vi "Write to CSV Test.vi"(8 "Error In":errorcluster) -> (0 "Error Out":errorcluster)   [LabVIEW 2023, in "Test.lvlib"]
uses:
  Test.lvlib
  <vilib>/addons/_JKI Toolkits/Caraya/classes/Assert/Assert Equal Value_Variant.vi
  <vilib>/addons/_JKI Toolkits/Caraya/classes/Assert/Assert.lvclass
  <vilib>/addons/_JKI Toolkits/Caraya/classes/Test/Test.lvclass
  File Path Operations/File and Path Operations.lvlib
panel:
  # "WRITE TO CSV TEST"
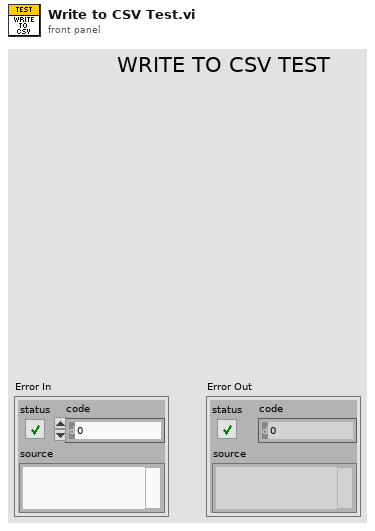
[diagram p1: front panel]
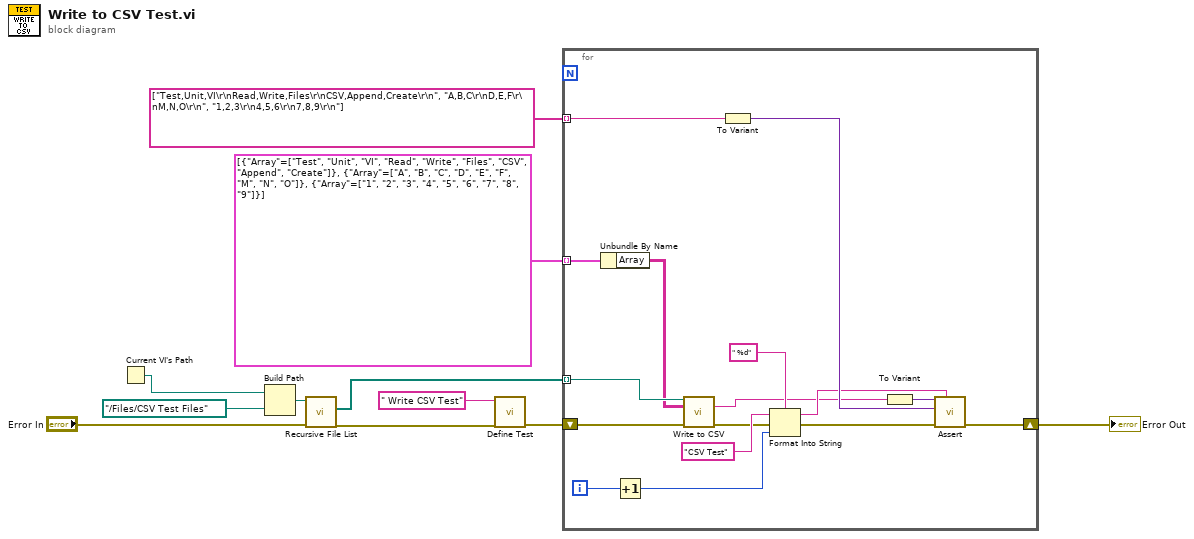
[diagram p0: block diagram]
diagram:
  n1 = Current VI's Path() -> (path=w5:path)
  n2 = Build Path(base path=w5, name or relative path=path "../Files/CSV Test Files") -> (appended path=w8:path)
  n3 = call <vilib>:"Recursive File List.vi"("error in (no error)"="Error In", "Folder Path"=w8) -> ("error out"=w7:errorcluster, "All Files in Dir"=w6:path[])  [unwired: 5 in, 3 out]
  n4 = call <vilib>:"Define Test.vi"("error in (no error)"=w7, "Label (VI Title)"=" Write CSV Test") -> ("error out"=w10:errorcluster)  [unwired: 8 in, 1 out]
  n5 = for {
    tunnel: w6 -> [w16] mode=indexing
    shift-right: [w19] -> w2
    shift-left: w10 -> [w18]
    tunnel: cluster{"Array":string[][]}[] [{"Array"=[["Test", "Unit", "VI"], ["Read", "Write", "Files"], ["CSV", "Append", "Create"]]}, {"Array"=[["A", "B", "C"], ["D", "E", "F"], ["M", "N", "O"]]}, {"Array"=[["1", "2", "3"], ["4", "5", "6"], ["7", "8", "9"]]}] -> [w15] mode=indexing
    tunnel: string[] ["Test,Unit,VI\r\nRead,Write,Files\r\nCSV,Append,Create\r\n", "A,B,C\r\nD,E,F\r\nM,N,O\r\n", "1,2,3\r\n4,5,6\r\n7,8,9\r\n"] ("File/Folder Name") -> [w13] mode=indexing
    i -> [w23]
    n6 = Unbundle By Name(w15) -> ("Array"=w14:string[][])
    n7 = Increment(x=w23) -> (x+1=w20:i32)
    n8 = call "Write to CSV.vi"("Path In"=w16, "Array In"=w14, "Error In"=w18) -> ("Log Data"=w12:string, "Error Out"=w17:errorcluster)  [unwired: 10 in, 1 out]
    n9 = To Variant(anything=w13) -> (Variant=w27:variant)
    n10 = Format Into String(format string=" %d", initial string="CSV Test" ("Label"), error in=w17, w20) -> (resulting string=w21:string, error out=w25:errorcluster)
    n11 = To Variant(anything=w12) -> (Variant=w26:variant)
    n12 = call-poly <vilib>:"Assert.vi"("Label"=w21, "error in (no error)"=w25, "Y"=w27, "X"=w26) -> ("error out"=w19:errorcluster)  [unwired: 6 in, 1 out]
  }
  "Error Out" <- w2
